vi "SUB_Write_GEN4_Init_data_V2_0_1.vi"(5 "Interval Time":enum16{"10ms", "33ms", "50ms"}(ring), 6 "PCAP zero information":T4 {"Sensor 8" format="%x"; "Sensor 7" format="%x"; "Sensor 6" format="%x"; "Sensor 5" format="%x"; "Sensor 4" format="%x"; "Sensor 3" format="%x"; "Sensor 2" format="%x"; "Sensor 1" format="%x"; "Packet ID" format="%x"}, 7 "Mode":T3, 8 "Connection Status":T1={"MAC Address"="F8:B8:54:EF:76:8D", "cnx handle"=0, "cnx flags"=5, "Address Type"=1, "Connection Interval (ms)"=8, "Timeout(ms)"=1000, "Latency"=0, "bonding handle"=255} {"Address Type" items=["Public", "Random"]}, 9 "Cal information":T5 {"Voltage L 2.8V" format="%x"; "Voltage H 2.8V" format="%x"; "Voltage L 3.1V" format="%x"; "Acc Z_L_Cal" format="%x"; "Voltage H 3.1V" format="%x"; "Gyro Z_L_Cal" format="%x"; "Gyro Z_H_Cal" format="%x"; "Gyro Y_L_Cal" format="%x"; "Gyro Y_H_Cal" format="%x"; "Gyro X_L_Cal" format="%x"; "Gyro X_H_Cal" format="%x"; "Acc Z_H_Cal" format="%x"; "Acc Y_L_Cal" format="%x"; "Acc Y_H_Cal" format="%x"; "Acc X_L_Cal" format="%x"; "Acc X_H_Cal" format="%x"; "Packet ID" format="%x"}, 10 "Device information":T6 {"Device Type L" format="%x"; "Device Type H" format="%x"; "Check sum" format="%x"; "Scale B" format="%x"; "Scale A" format="%x"; "Manufacturer Lot ID 4" format="%x"; "Manufacturer Lot ID 3" format="%x"; "Manufacturer Lot ID 2" format="%x"; "Manufacturer Lot ID 1" format="%x"; "Day" format="%x"; "Month" format="%x"; "Year" format="%x"; "Device ID 4" format="%x"; "Device ID 3" format="%x"; "Device ID 2" format="%x"; "Device ID 1" format="%x"; "Packet ID" format="%x"}, 11 "Port-act 1":refnum<visa-resource-name>="COM8") -> ()   [LabVIEW 2015]
uses:
  Cluster Type/Device information.ctl
  Cluster Type/Cal information.ctl
  Cluster Type/PCAP zero information.ctl
  Type definition/write_mode.ctl
  Lib_Bled112 toolkit/type_def/connection_status_bundle.ctl
  Lib_Bled112 toolkit/type_def/address_type.ctl
  Lib_Bled112 toolkit/ble_functions/ble_write_by_handle_uint8array.vi
panel:
  in  "Delay(ms)":u32=3
  # "(Device Type is divided 1byte)"
  # "=> Sensor Offset Valure"
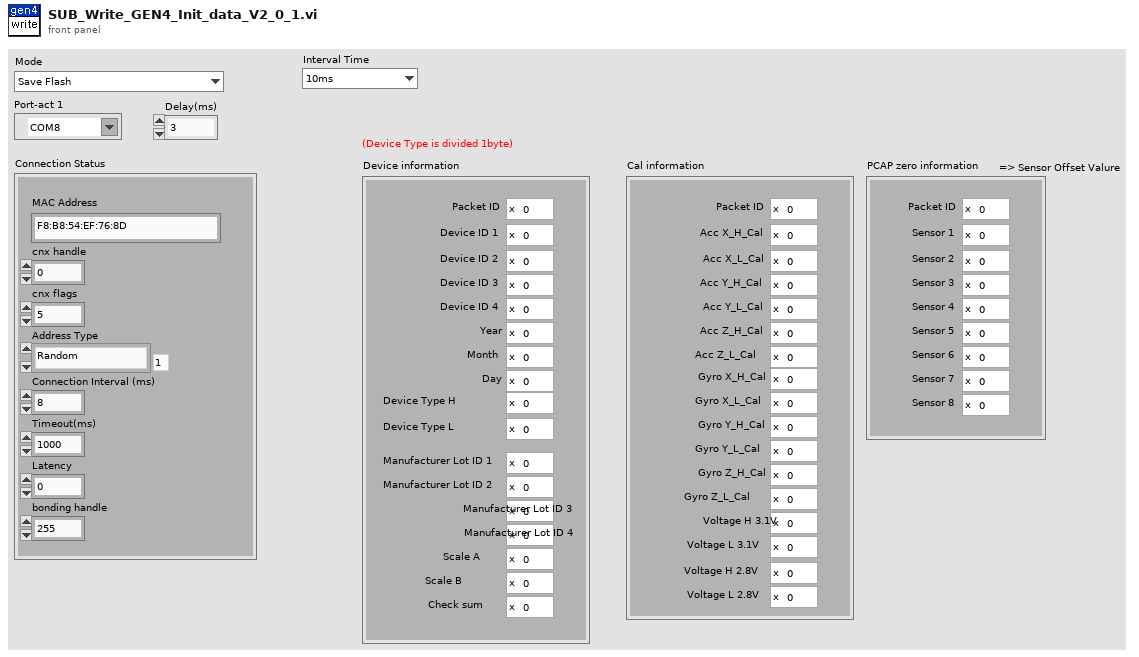
[diagram p1: front panel]
types:
  T1 = typedef "connection_status_bundle.ctl" = cluster{"MAC Address":string, "cnx handle":u8, "cnx flags":u8, "Address Type":T2, "Connection Interval (ms)":u16, "Timeout(ms)":u16, "Latency":u16, "bonding handle":u8}
  T2 = typedef "address_type.ctl" = u8
  T3 = typedef "write_mode.ctl" = enum16{"Save Flash", "Visa save", "Interval Change"}
  T4 = typedef "PCAP zero information.ctl" = cluster{"Packet ID":u8, "Sensor 1":u16, "Sensor 2":u16, "Sensor 3":u16, "Sensor 4":u16, "Sensor 5":u16, "Sensor 6":u16, "Sensor 7":u16, "Sensor 8":u16}
  T5 = typedef "Cal information.ctl" = cluster{"Packet ID":u8, "Acc X_H_Cal":u8, "Acc X_L_Cal":u8, "Acc Y_H_Cal":u8, "Acc Y_L_Cal":u8, "Acc Z_H_Cal":u8, "Acc Z_L_Cal":u8, "Gyro X_H_Cal":u8, "Gyro X_L_Cal":u8, "Gyro Y_H_Cal":u8, "Gyro Y_L_Cal":u8, "Gyro Z_H_Cal":u8, "Gyro Z_L_Cal":u8, "Voltage H 3.1V":u8, "Voltage L 3.1V":u8, "Voltage H 2.8V":u8, "Voltage L 2.8V":u8}
  T6 = typedef "Device information.ctl" = cluster{"Packet ID":u8, "Device ID 1":u8, "Device ID 2":u8, "Device ID 3":u8, "Device ID 4":u8, "Year":u8, "Month":u8, "Day":u8, "Device Type H":u8, "Device Type L":u8, "Manufacturer Lot ID 1":u8, "Manufacturer Lot ID 2":u8, "Manufacturer Lot ID 3":u8, "Manufacturer Lot ID 4":u8, "Scale A":u8, "Scale B":u8, "Check sum":u8}
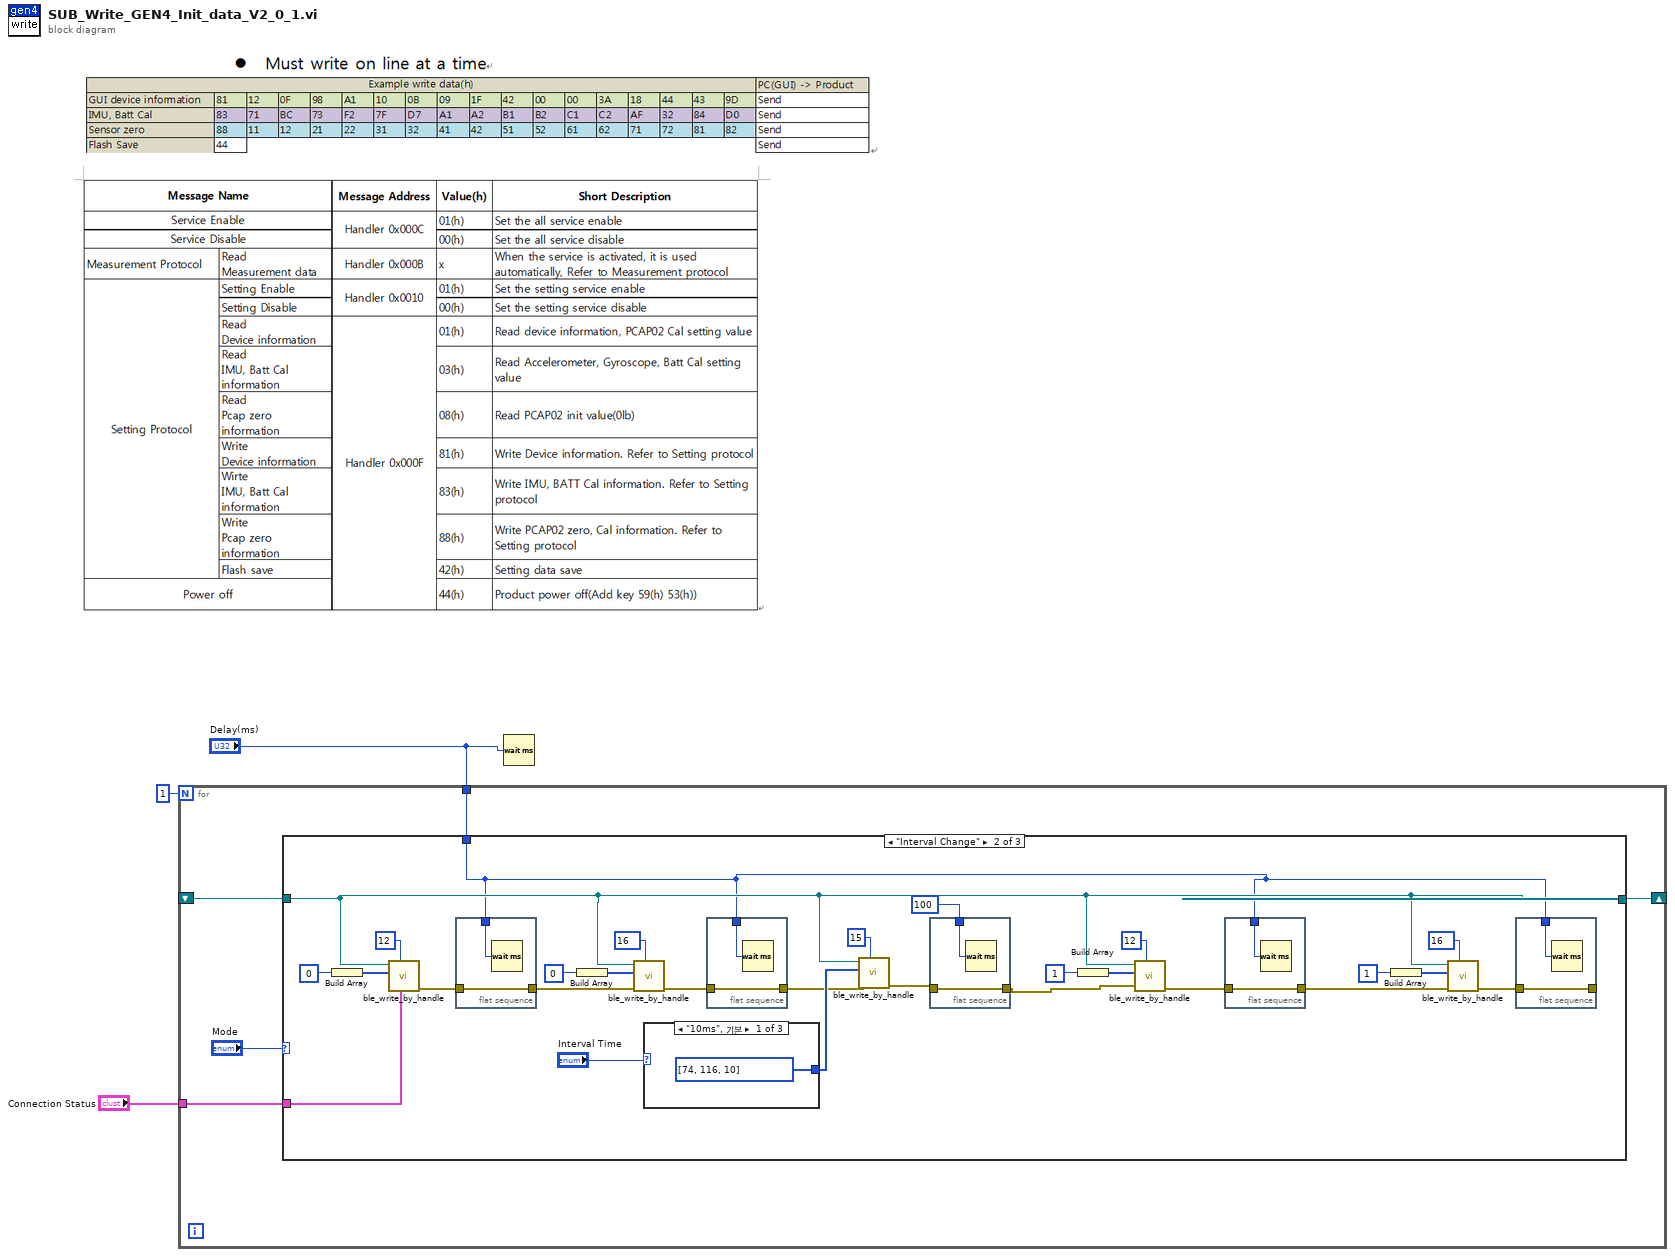
[diagram p0: block diagram]
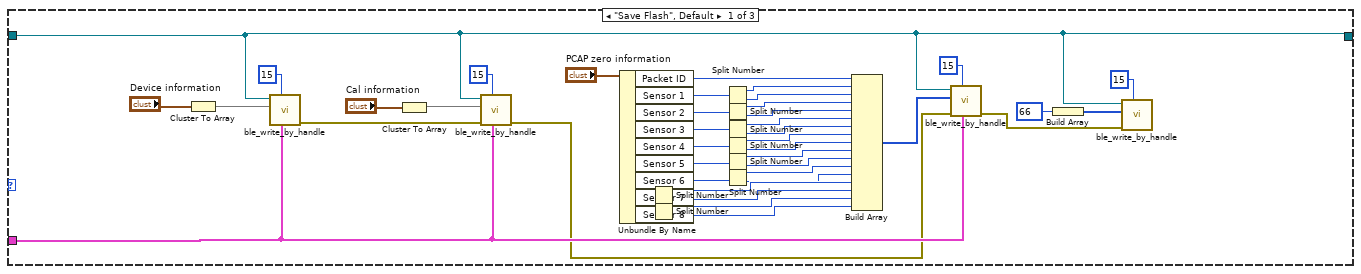
[diagram p2: hidden frame]
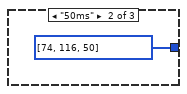
[diagram p3: hidden frame]
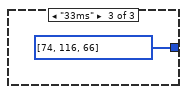
[diagram p4: hidden frame]
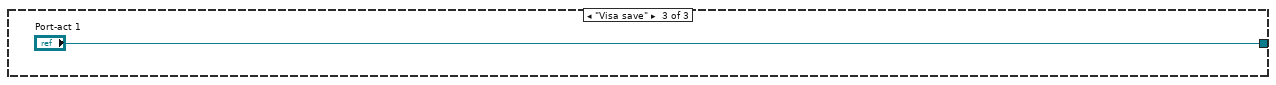
[diagram p5: hidden frame]
diagram:
  n1 = for {
    N: 1 -> [_]
    shift-right: [w7] -> _
    shift-left: _ -> [w6]
    tunnel: "Connection Status" -> [w5]
    tunnel: "Delay(ms)" -> [w4]
    n2 = case shown="\"Interval Change\"" "Mode" {
      tunnel: [w9 w64 "Port-act 1"] -> w7
      tunnel: w6 -> [w9 w64 _]
      tunnel: w5 -> [w15 w77 _]
      tunnel: w4 -> [_ w52 _]
      frame "Save Flash", Default {
        n3 = Cluster To Array(cluster="Device information") -> (array=w48:u8[])
        n4 = call-poly "ble_write_by_handle.vi"("Connection Status"=w15, "Handle"=u16 15, "data (uint8array)"=w48, "COM Bluegiga in"=w9) -> ("error out"=w44:errorcluster)  [unwired: 6 in, 1 out]
        n5 = Cluster To Array(cluster="Cal information") -> (array=w45:u8[])
        n6 = call-poly "ble_write_by_handle.vi"("Connection Status"=w15, "Handle"=u16 15, "error in (no error)"=w44, "data (uint8array)"=w45, "COM Bluegiga in"=w9) -> ("error out"=w14:errorcluster)  [unwired: 5 in, 1 out]
        n7 = Unbundle By Name("PCAP zero information") -> ("Packet ID"=w26:u8, "Sensor 1"=w18:u16, "Sensor 2"=w19:u16, "Sensor 3"=w20:u16, "Sensor 4"=w21:u16, "Sensor 5"=w22:u16, "Sensor 6"=w23:u16, "Sensor 7"=w24:u16, "Sensor 8"=w25:u16)
        n8 = Split Number(x=w24) -> (hi(x)=w39:u8, lo(x)=w40:u8)
        n9 = Split Number(x=w25) -> (hi(x)=w41:u8, lo(x)=w42:u8)
        n10 = Split Number(x=w18) -> (hi(x)=w27:u8, lo(x)=w28:u8)
        n11 = Split Number(x=w19) -> (hi(x)=w29:u8, lo(x)=w30:u8)
        n12 = Split Number(x=w20) -> (hi(x)=w31:u8, lo(x)=w32:u8)
        n13 = Split Number(x=w21) -> (hi(x)=w33:u8, lo(x)=w34:u8)
        n14 = Split Number(x=w22) -> (hi(x)=w35:u8, lo(x)=w36:u8)
        n15 = Split Number(x=w23) -> (hi(x)=w37:u8, lo(x)=w38:u8)
        n16 = Build Array(w26, w27, w28, w29, w30, w31, w32, w33, w34, w35, w36, w37, w38, w39, w40, w41, w42) -> (w16:u8[])
        n17 = call-poly "ble_write_by_handle.vi"("Connection Status"=w15, "Handle"=u16 15, "error in (no error)"=w14, "data (uint8array)"=w16, "COM Bluegiga in"=w9) -> ("error out"=w10:errorcluster)  [unwired: 5 in, 1 out]
        n18 = Build Array(u16 66 ("Handle")) -> (w11:u16[])
        n19 = call-poly "ble_write_by_handle.vi"("Handle"=u16 15, "error in (no error)"=w10, "data (uint8array)"=w11, "COM Bluegiga in"=w9) -> ()  [unwired: 6 in, 2 out]
      }
      frame "Interval Change" {
        n20 = Build Array(u16 0 ("Handle")) -> (w75:u16[])
        n21 = call-poly "ble_write_by_handle.vi"("Connection Status"=w77, "Handle"=u16 12, "data (uint8array)"=w75, "COM Bluegiga in"=w64) -> ("error out"=w60:errorcluster)  [unwired: 6 in, 1 out]
        n22 = flat-sequence {
          tunnel: w52 -> [w88]
          tunnel: [w87] -> w61
          tunnel: w60 -> [w87]
          frame #0 {
            n23 = Wait (ms)(milliseconds to wait=w88) -> ()  [unwired: 1 out]
          }
        }
        n24 = Build Array(u16 0 ("Handle")) -> (w74:u16[])
        n25 = call-poly "ble_write_by_handle.vi"("Handle"=u16 16, "error in (no error)"=w61, "data (uint8array)"=w74, "COM Bluegiga in"=w64) -> ("error out"=w59:errorcluster)  [unwired: 6 in, 1 out]
        n26 = case shown="\"10ms\", 기본" "Interval Time" {
          tunnel: [u8[] [74, 116, 10] u8[] [74, 116, 50] u8[] [74, 116, 66]] -> w62
          frame "10ms", Default {
          }
          frame "50ms" {
          }
          frame "33ms" {
          }
        }
        n27 = flat-sequence {
          tunnel: w52 -> [w86]
          tunnel: [w85] -> w58
          tunnel: w59 -> [w85]
          frame #0 {
            n28 = Wait (ms)(milliseconds to wait=w86) -> ()  [unwired: 1 out]
          }
        }
        n29 = call-poly "ble_write_by_handle.vi"("Handle"=u16 15, "error in (no error)"=w58, "data (uint8array)"=w62, "COM Bluegiga in"=w64) -> ("error out"=w57:errorcluster)  [unwired: 6 in, 1 out]
        n30 = flat-sequence {
          tunnel: u32 100 ("대기 시간(ms)") -> [w84]
          tunnel: [w83] -> w56
          tunnel: w57 -> [w83]
          frame #0 {
            n31 = Wait (ms)(milliseconds to wait=w84) -> ()  [unwired: 1 out]
          }
        }
        n32 = Build Array(u16 1 ("Handle")) -> (w68:u16[])
        n33 = call-poly "ble_write_by_handle.vi"("Handle"=u16 12, "error in (no error)"=w56, "data (uint8array)"=w68, "COM Bluegiga in"=w64) -> ("error out"=w55:errorcluster)  [unwired: 6 in, 1 out]
        n34 = flat-sequence {
          tunnel: w52 -> [w82]
          tunnel: [w81] -> w54
          tunnel: w55 -> [w81]
          frame #0 {
            n35 = Wait (ms)(milliseconds to wait=w82) -> ()  [unwired: 1 out]
          }
        }
        n36 = Build Array(u16 1 ("Handle")) -> (w69:u16[])
        n37 = call-poly "ble_write_by_handle.vi"("Handle"=u16 16, "error in (no error)"=w54, "data (uint8array)"=w69, "COM Bluegiga in"=w64) -> ("error out"=w53:errorcluster)  [unwired: 6 in, 1 out]
        n38 = flat-sequence {
          tunnel: w52 -> [w80]
          tunnel: [w79] -> _
          tunnel: w53 -> [w79]
          frame #0 {
            n39 = Wait (ms)(milliseconds to wait=w80) -> ()  [unwired: 1 out]
          }
        }
      }
      frame "Visa save" {
      }
    }
  }
  n40 = Wait (ms)(milliseconds to wait="Delay(ms)") -> ()  [unwired: 1 out]
